vi "from_vi_name_and_path.vi"(5 "type":refnum<class "HierarchyNode.lvclass">, 8 "error in (no error)":errorcluster, 9 "vi_path":path, 10 "vi_name":string) -> (0 "error out":errorcluster, 3 "VINode out":refnum<class "HierarchyNode.lvclass">)   [LabVIEW 2020, in "vi-hierarchy.lvlib" / "HierarchyNode.lvclass"]
uses:
  HierarchyNode.lvclass
  C:/Projects/labview-project-load-tools/source/submodules/graph-api-labview/source/api/Node/Node.lvclass
  HierarchyNode.lvclass/HierarchyNode.ctl
  api/Node/Node.lvclass
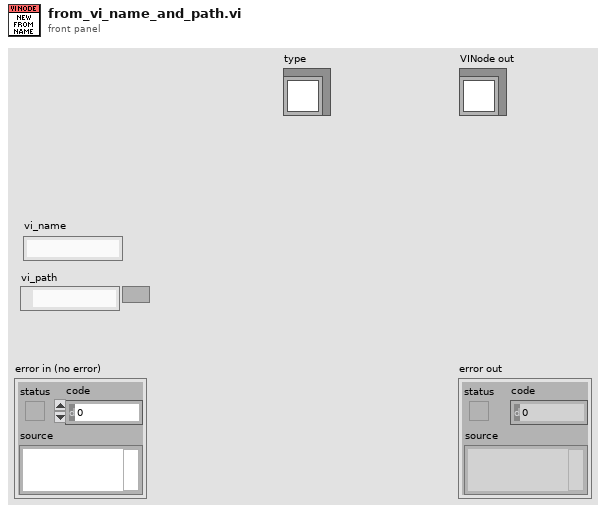
[diagram p1: front panel]
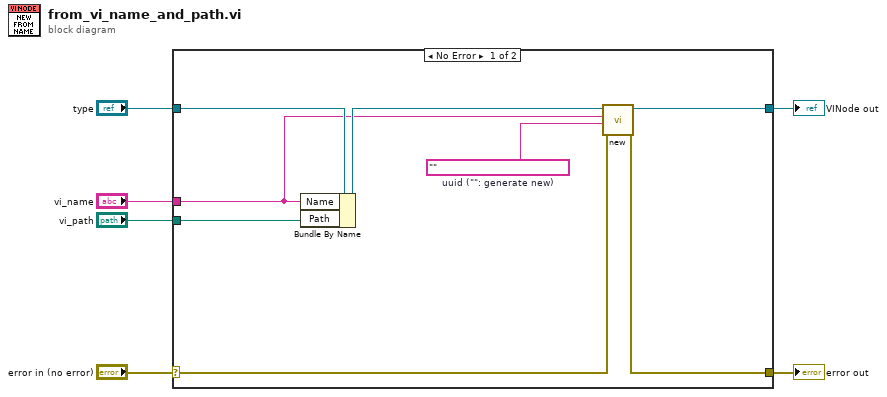
[diagram p0: block diagram]
diagram:
  n1 = case shown="No Error" "error in (no error)" {
    selector: "error in (no error)" -> [w11 w16]
    tunnel: [w10 w16] -> w5
    tunnel: [w12 w15] -> w3
    tunnel: "type" -> [w14 w15]
    tunnel: "vi_name" -> [w7 _]
    tunnel: "vi_path" -> [w9 _]
    frame No Error {
      w8 = ""  # uuid ("": generate new)
      n2 = Bundle By Name(cluster=w14, "Name"=w7, "Path"=w9) -> (w13:refnum<class "HierarchyNode.lvclass">)
      n3 = call "new.vi"("error in (no error)"=w11, "guid (\"\": generate new)"=w8, "label (\"\")"=w7, "Node in"=w13) -> ("error out"=w10:errorcluster, "Node out"=w12:refnum<class "HierarchyNode.lvclass">)  [unwired: 6 in]
    }
    frame Error {
    }
  }
  "error out" <- w5
  "VINode out" <- w3
